vi "SD-Match Regular Expression SaveForPrev85To82.vi"(10 "Version-State Cluster In":T1, 11 "XRef":refnum<vi>) -> (0 "Custom Label":string, 1 "Custom Warning To Issue":string, 2 "Version-State Cluster Out":T1, 3 "Action":T2)   [LabVIEW 2020, in "SD-Match Regular Expression.xnode"]
uses:
  SD-Match Regular Expression.xnode
  SD-SFPChangeStateAction.ctl
  SD-NI_XSFPSupport.lvlib
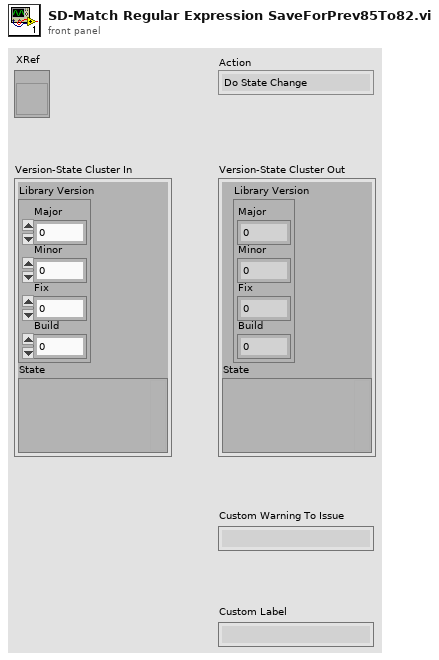
[diagram p1: front panel]
types:
  T1 = cluster{"Library Version":cluster{"Major":u16, "Minor":u16, "Fix":u16, "Build":u16}, "State":variant}
  T2 = typedef "SD-NI_XSFPSupport.lvlib/SD-SFPChangeStateAction.ctl" = enum32{"Do State Change", "Replace With Label", "Fail SFP"}
  T3 = cluster{"Major":u16, "Minor":u16, "Fix":u16, "Build":u16}
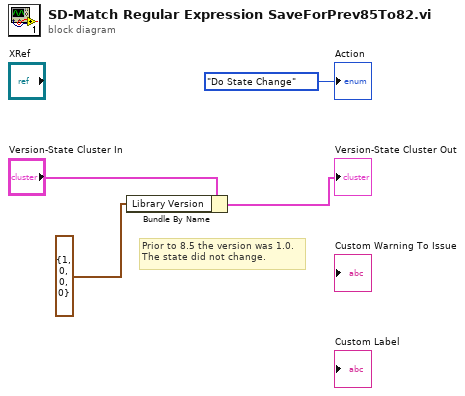
[diagram p0: block diagram]
diagram:
  # "Prior to 8.5 the version was 1.0.\nThe state did not change."
  n1 = Bundle By Name(cluster="Version-State Cluster In", "Library Version"=T3 {"Major"=1, "Minor"=0, "Fix"=0, "Build"=0}) -> (→"Version-State Cluster Out":T1)
  "Action" <- SD-SFPChangeStateAction."Do State Change" ("Action")
